vi "Main.vi"() -> ()   [LabVIEW 2025, in "IT-M3900C.lvlib"]
uses:
  IT-M3900C.lvlib
  States Enum.ctl
  Data.ctl
  PS Settings Cluster.ctl
panel:
  out "XY Graph":cluster{timestamp[], dbl[]}[](graph)
  in  "Save":bool
  in  "Test Settings":T1
  in  "Supply Settings":T2={"Repeat"=0, "Terminate Type"=0, "Save File"=1, "Type"=0, "Normal Current(A)"=0.0, "Normal Voltage(V)"=0.0} {"Normal Voltage(V)" min=0.0; "Type" items=["Current", "Voltage"]; "Save File" min=1 max=10; "Terminate Type" items=["Normal", "Last", "Off"]; "Repeat" min=0}
  in  "Current Setpoint":dbl format="%#_g A"
  in  "Set":bool
  in  "Voltage Setpoint":dbl format="%#_g V"
  in  "Enable":bool
  in  "Run":bool
  in  "COM Port":refnum<visa-resource-name>
  out "error out":errorcluster
  in  "error in":errorcluster
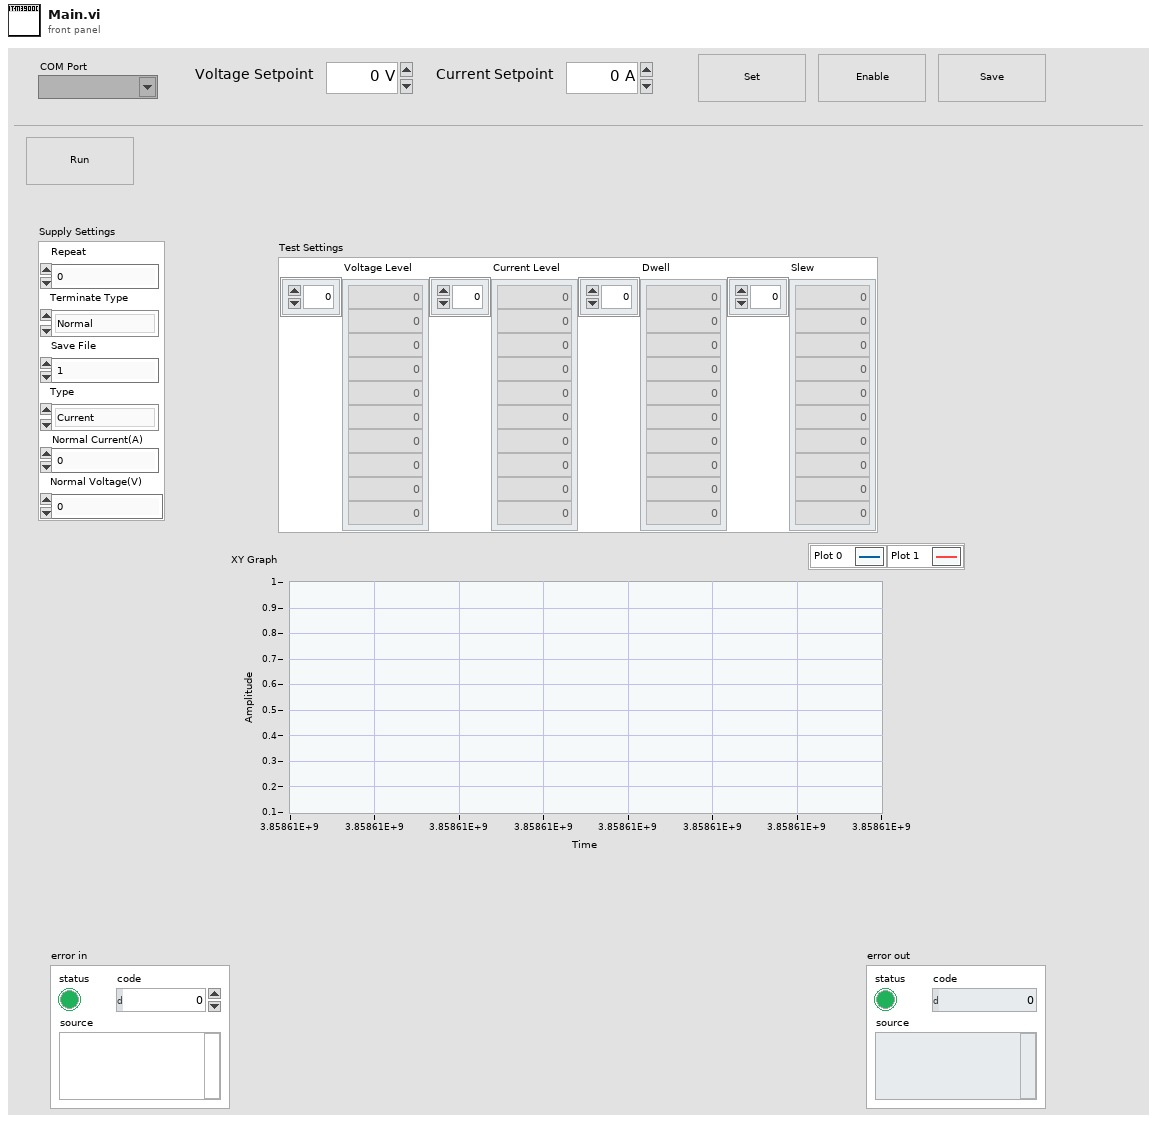
[diagram p1: front panel]
types:
  T1 = cluster{"Voltage Level":dbl[], "Current Level":dbl[], "Dwell":dbl[], "Slew":dbl[]}
  T2 = cluster{"Repeat":i32, "Terminate Type":u16, "Save File":i32, "Type":u16, "Normal Current(A)":dbl, "Normal Voltage(V)":dbl}
  T3 = typedef "IT-M3900C.lvlib/Data.ctl" = cluster{"PS Settings":T4, "Reports Ref":refnum<file>, "Test Settings Ref":refnum<file>, "Test Settings":cluster{"Voltage Level":dbl[], "Current Level":dbl[], "Dwell":dbl[], "Slew":dbl[]}}
  T4 = typedef "IT-M3900C.lvlib/PS Settings Cluster.ctl" = cluster{"COM Port":refnum<visa-resource-name>, "IT Ref":refnum<visa-resource-name>}
  T5 = typedef "IT-M3900C.lvlib/States Enum.ctl" = enum16{"Initialize", "Idle", "Prep Test", "Run", "Wait for Run", "Results", "Exit"}
  T6 = cluster{"Baud Rate":u32, "Parity":u16, "Data Bits":u16, "Stop Bits":u16, "Flow Control":u16}
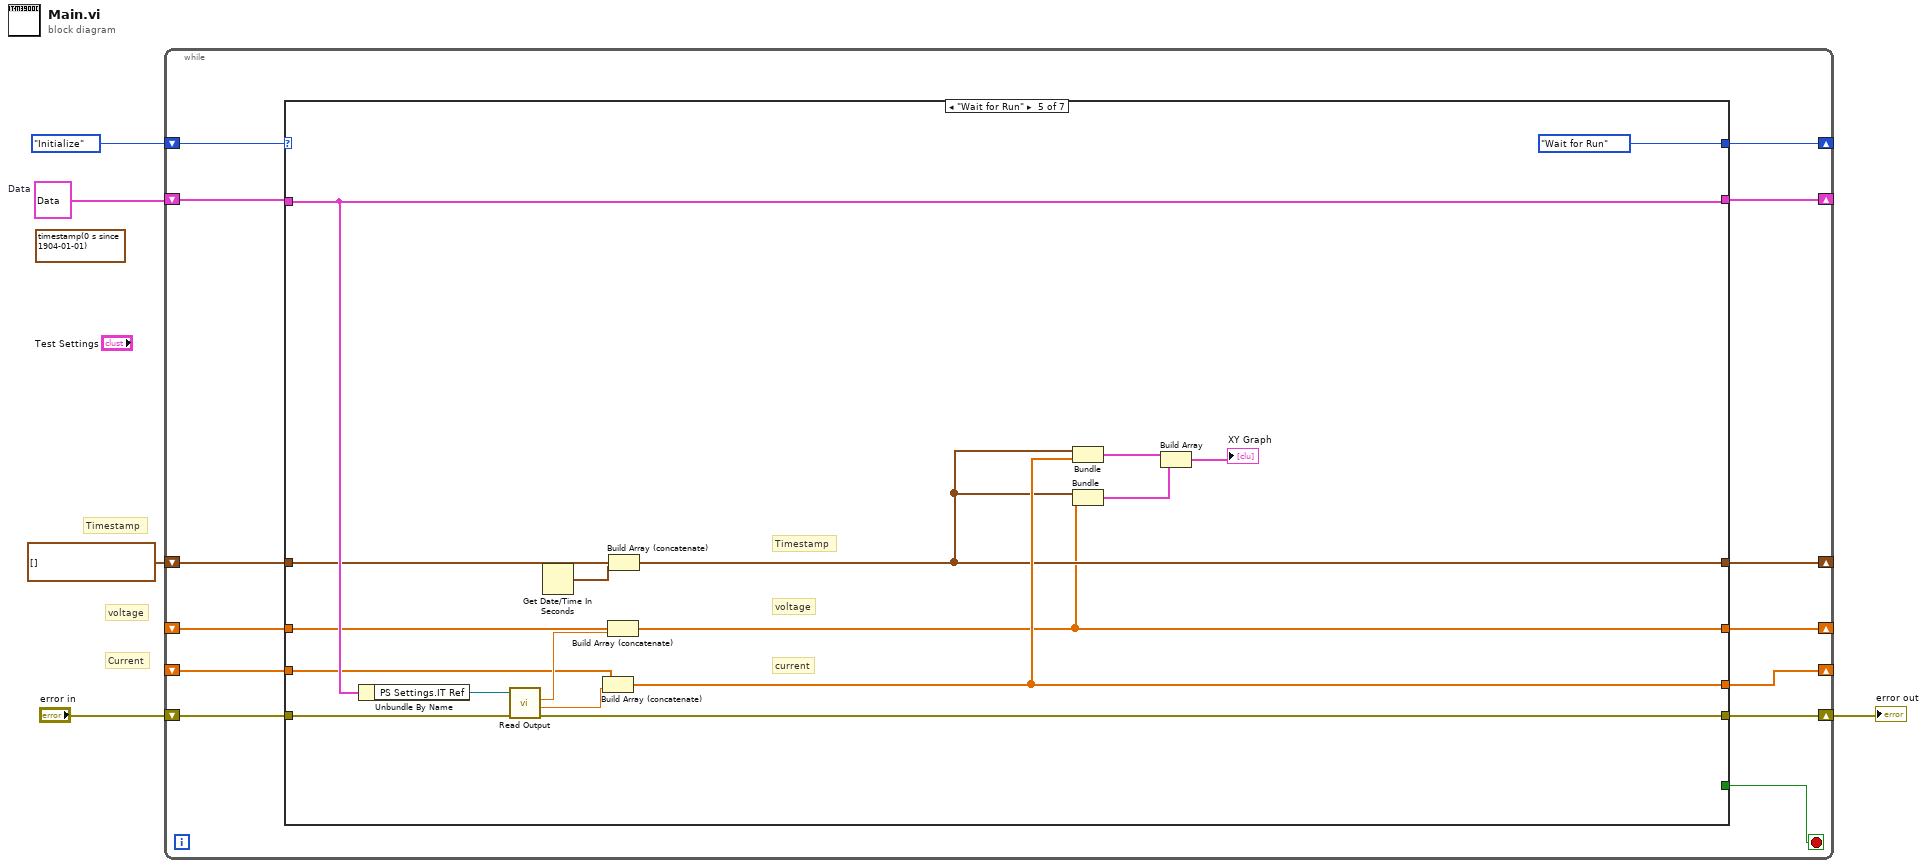
[diagram p0: block diagram]
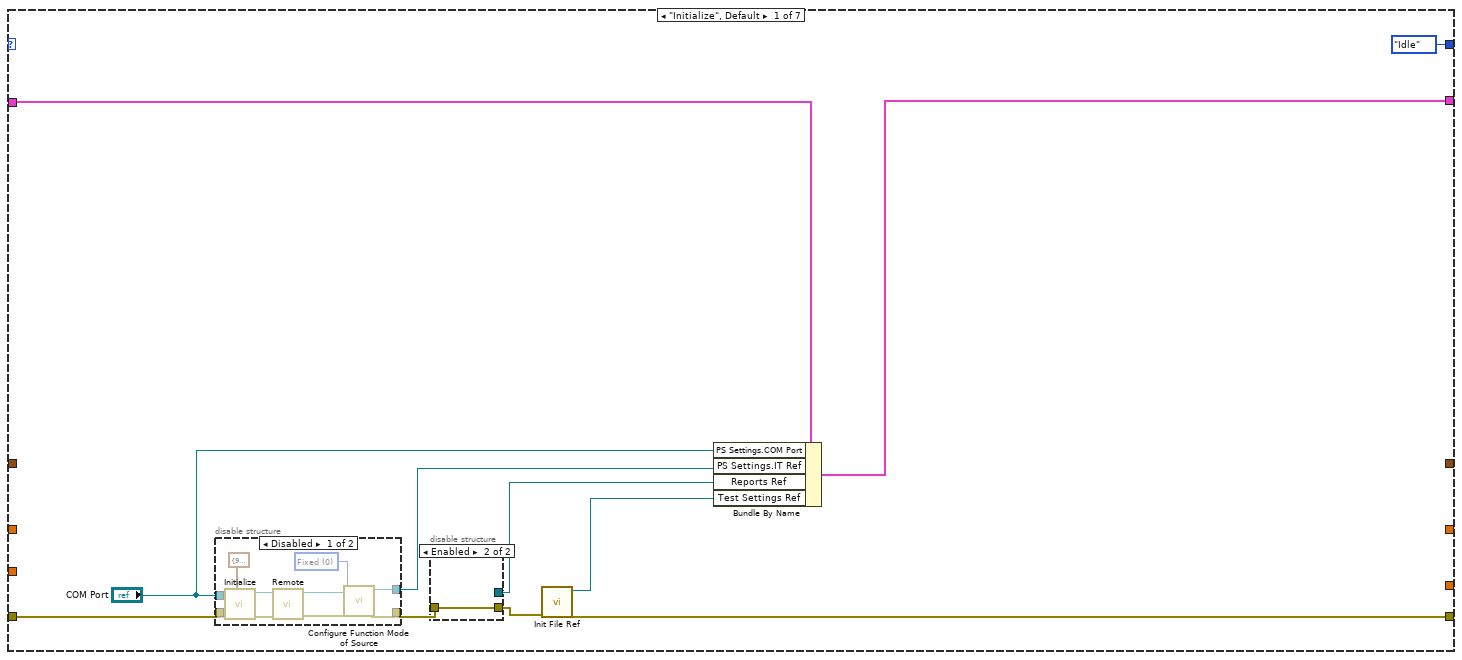
[diagram p2: hidden frame]
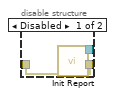
[diagram p3: hidden frame]
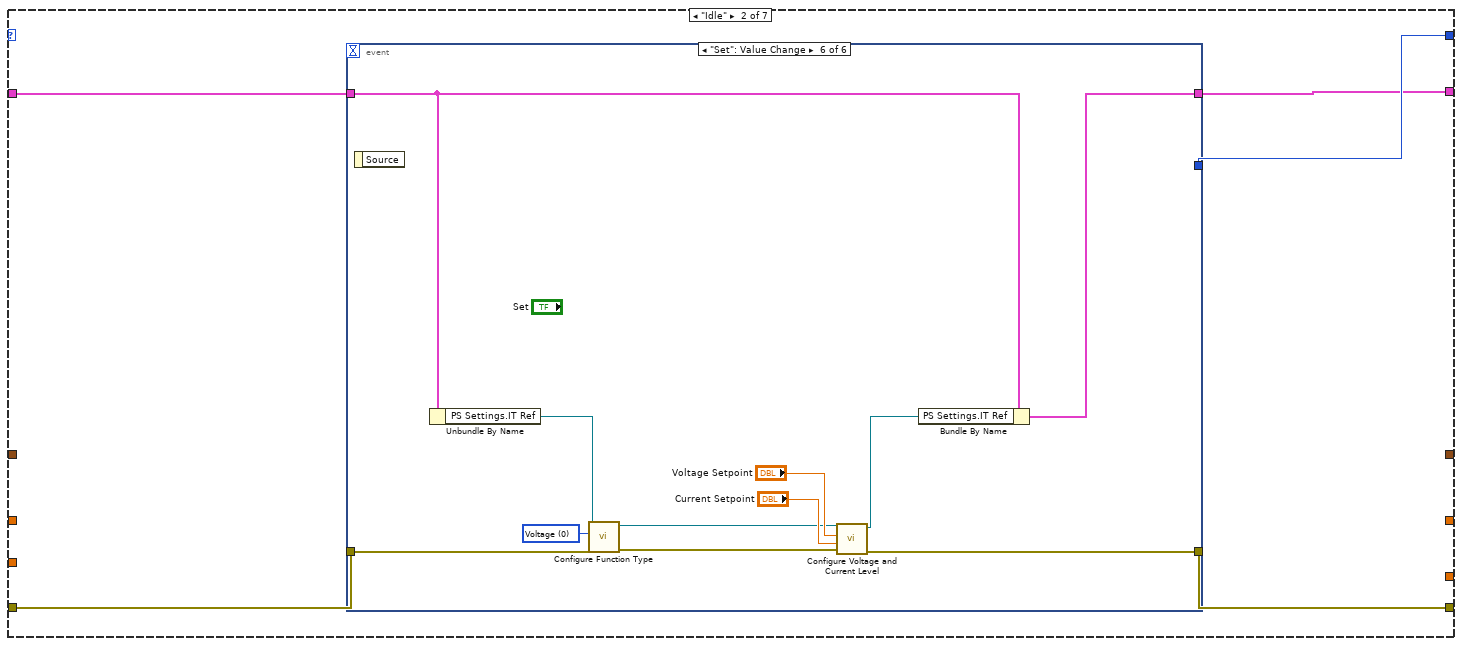
[diagram p5: hidden frame]
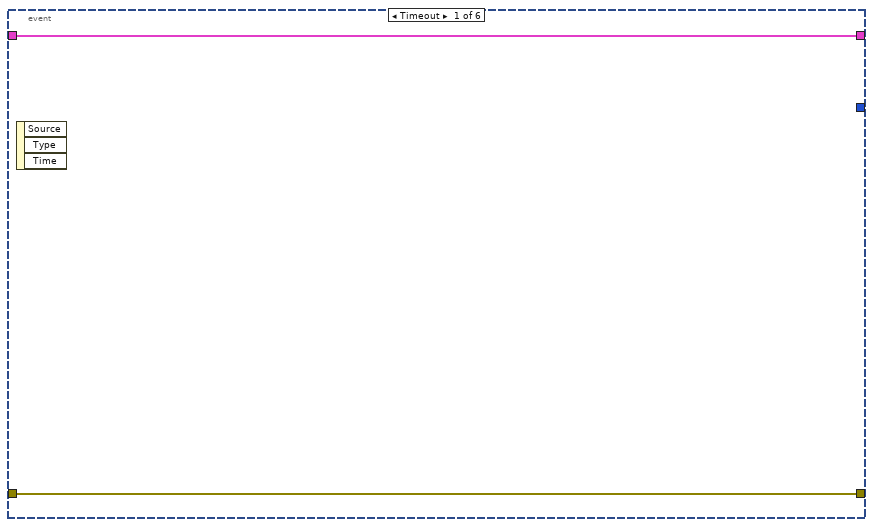
[diagram p6: hidden frame]
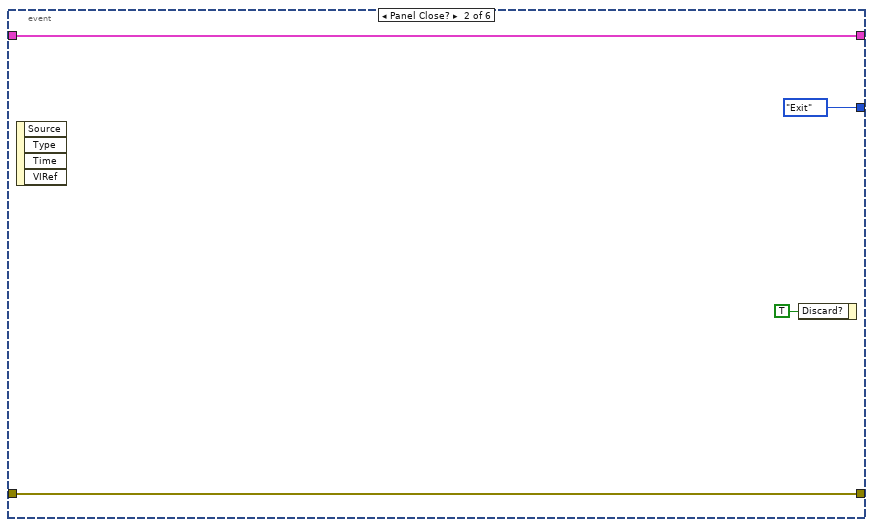
[diagram p7: hidden frame]
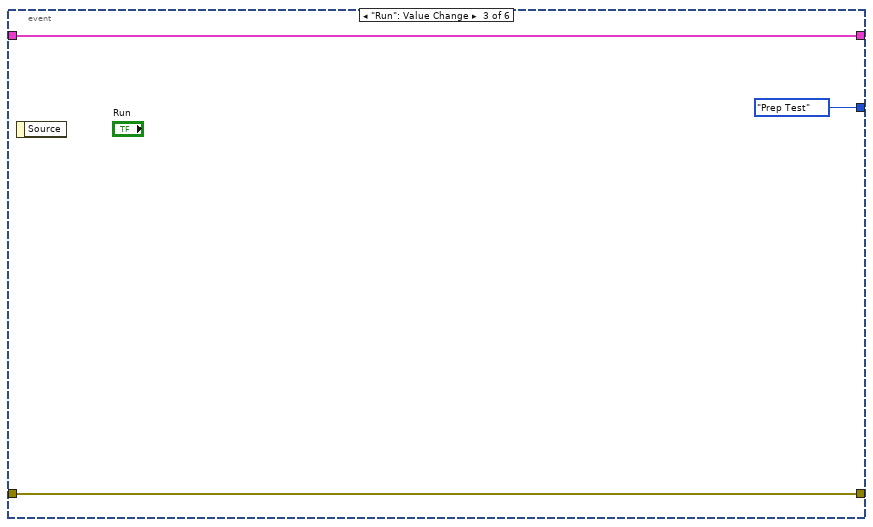
[diagram p8: hidden frame]
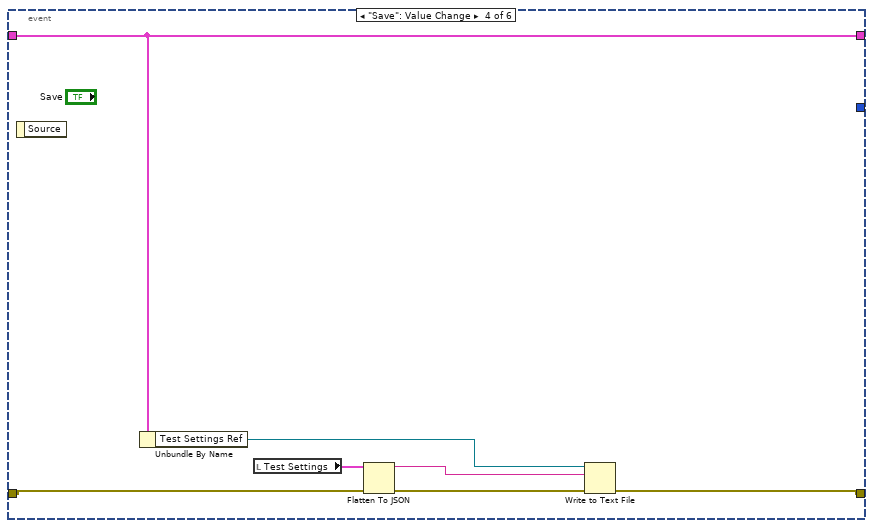
[diagram p9: hidden frame]
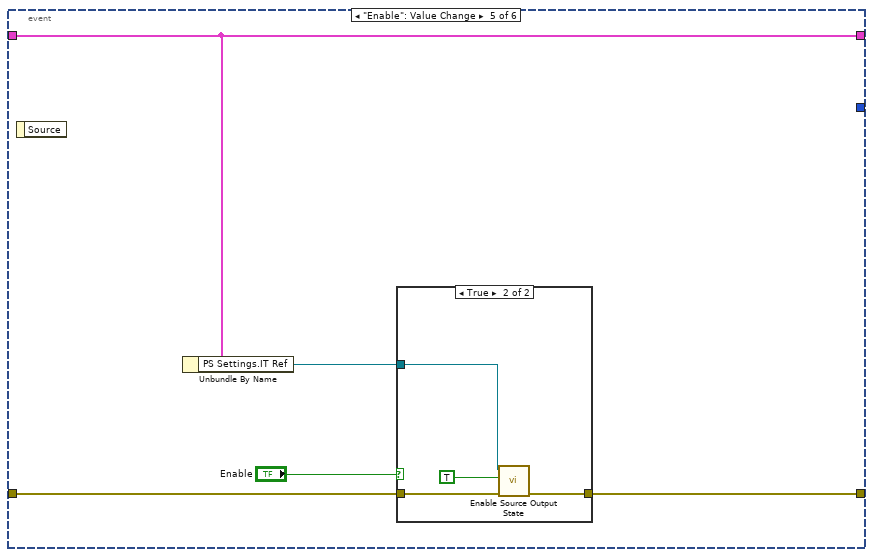
[diagram p10: hidden frame]
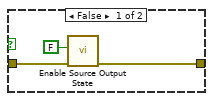
[diagram p11: hidden frame]
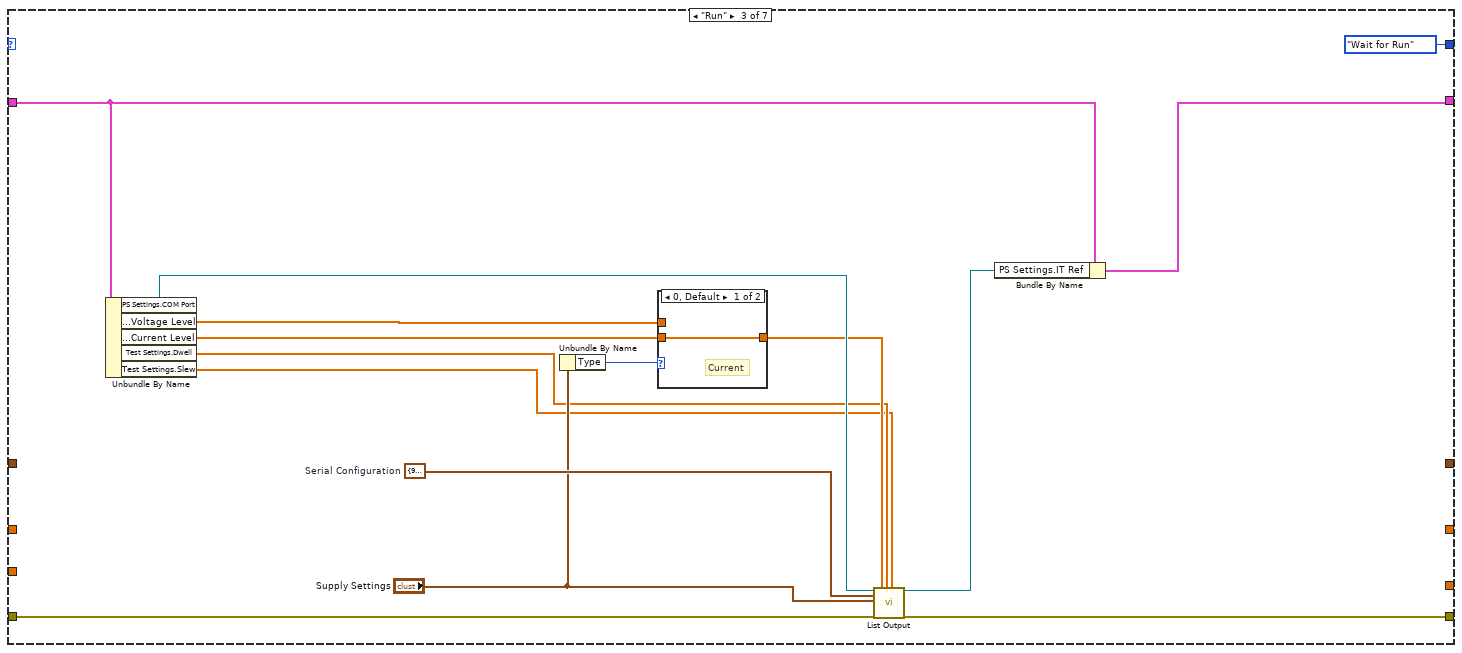
[diagram p12: hidden frame]
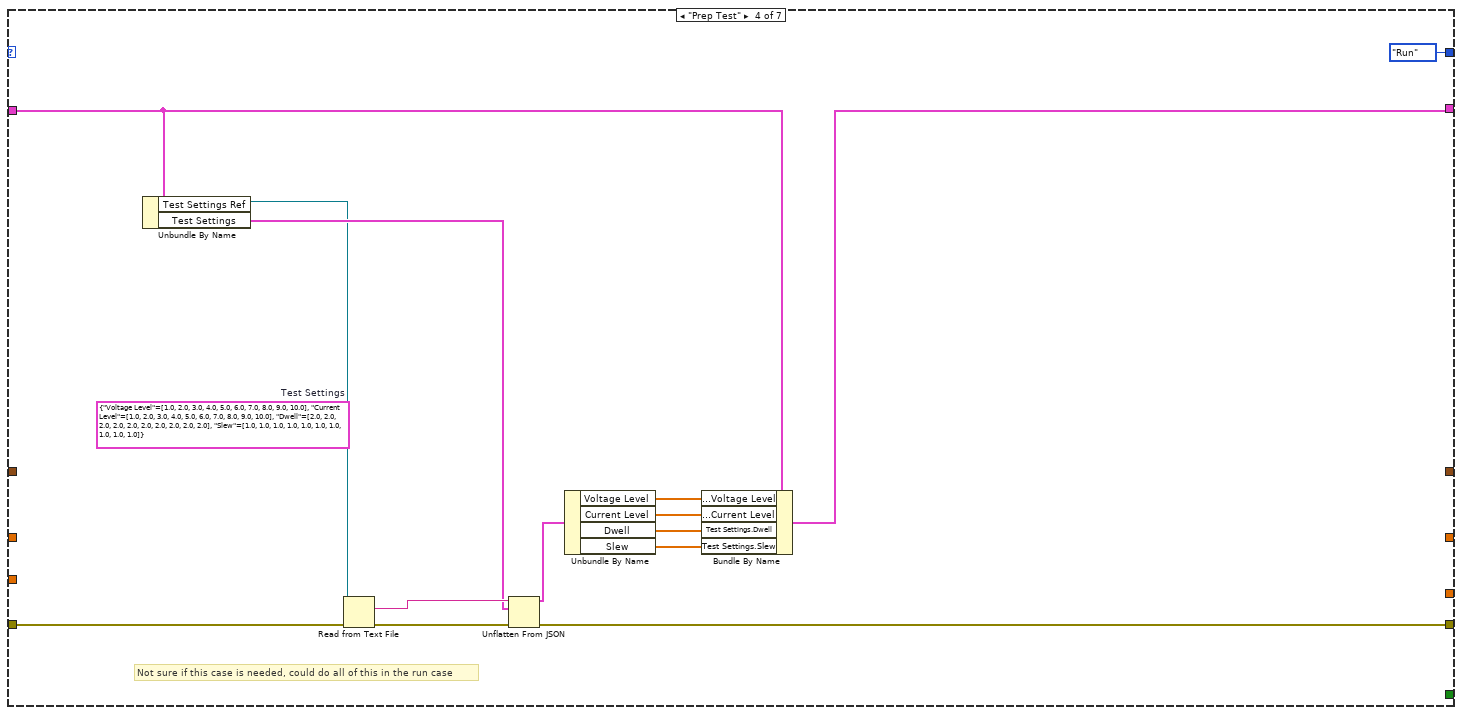
[diagram p14: hidden frame]
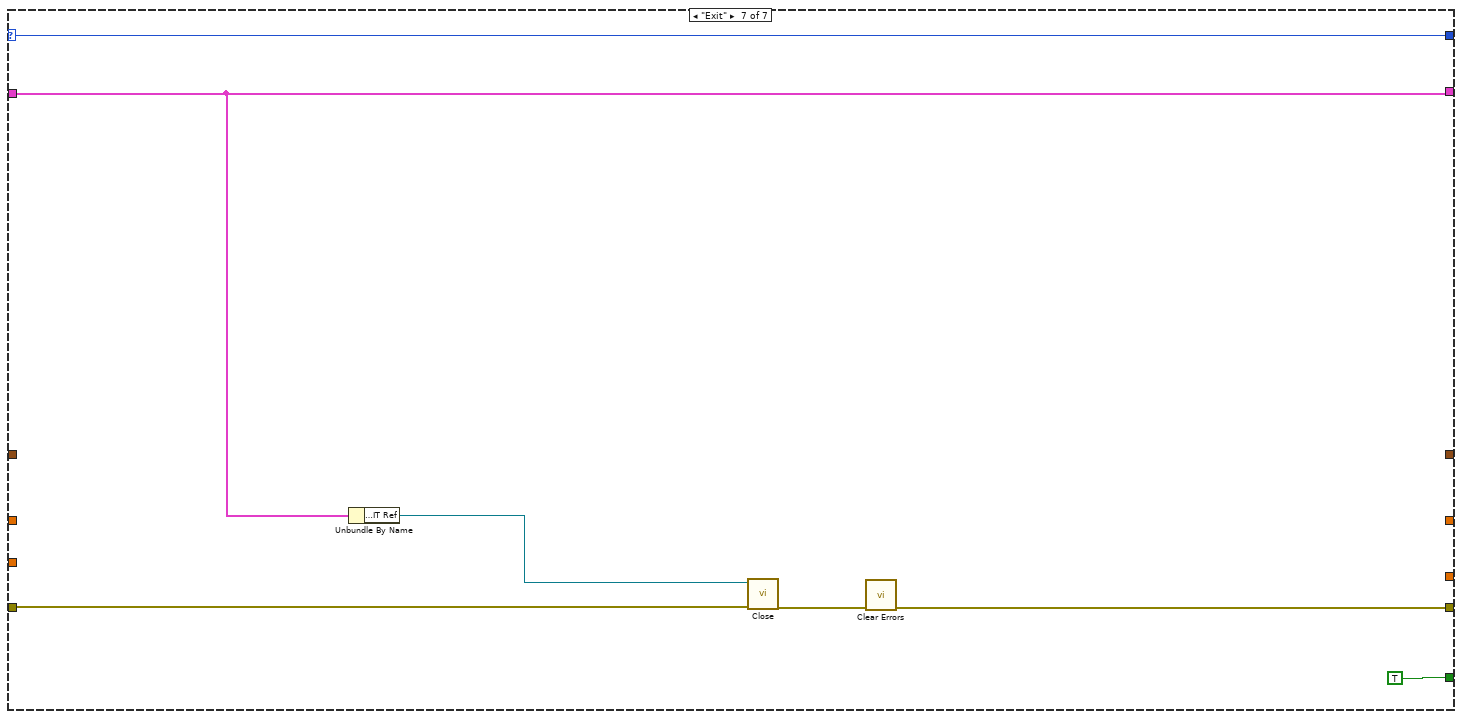
[diagram p16: hidden frame]
diagram:
  (unwired) timestamp(0 s since 1904-01-01) ("seconds since 1Jan1904")
  w2 = T3 {"PS Settings"={"COM Port"="", "IT Ref"=""}, "Reports Ref"=refnum, "Test Settings Ref"=refnum, "Test Settings"={"Voltage Level"=[], "Current Level"=[], "Dwell"=[], "Slew"=[]}}  # Data
  # "Current"
  # "Timestamp"
  # "voltage"
  n1 = while {
    shift-right: [w17] -> _
    shift-left: States_Enum."Initialize" ("States") -> [w18]
    shift-right: [w14] -> w3
    shift-left: "error in" -> [w15]
    shift-right: [w13] -> _
    shift-left: w2 -> [w12]
    shift-right: [w11] -> _
    shift-left: _ -> [w10]
    shift-right: [w9] -> _
    shift-left: timestamp[] [] -> [w8]
    shift-right: [w7] -> _
    shift-left: _ -> [w6]
    stop <- w16 stop-if-true
    n2 = case shown="\"Wait for Run\"" w18 {
      selector: w18 -> [_ _ _ _ _ _ w145]
      tunnel: [States_Enum."Idle" ("States") w48 States_Enum."Wait for Run" ("States") States_Enum."Run" ("States") States_Enum."Wait for Run" ("States") _ w145] -> w17
      tunnel: [_ _ _ _ _ _ TRUE] -> w16
      tunnel: w15 -> [w26 w49 w103 w118 w136 w138 w141]
      tunnel: [w25 w45 w102 w116 w135 w138 w139] -> w14
      tunnel: w12 -> [w29 w47 w90 w112 w134 w137 w143]
      tunnel: [w28 w46 w91 w113 w134 w137 w143] -> w13
      tunnel: [_ _ _ _ w123 _ _] -> w11
      tunnel: w10 -> [_ _ _ _ w131 _ _]
      tunnel: [_ _ _ _ w124 _ _] -> w9
      tunnel: w8 -> [_ _ _ _ w129 _ _]
      tunnel: [_ _ _ _ w126 _ _] -> w7
      tunnel: w6 -> [_ _ _ _ w127 _ _]
      frame "Initialize", Default {
        n3 = disable-structure shown="Disabled" {
          disable-tunnel: w26 -> [w43 w44]
          disable-tunnel: [w39 w44] -> w23
          disable-tunnel: [w37 _] -> w22
          disable-tunnel: "COM Port" -> [w34 _]
          frame Disabled {
            w36 = u16 0 items=["Fixed", "List", "Battery", "Solar", "CarProfile", "Fuel", "Step"] ("Mode")
            n4 = call "Initialize.vi"("Serial Configuration"=T6 {"Baud Rate"=9600, "Parity"=0, "Data Bits"=8, "Stop Bits"=10, "Flow Control"=0}, "error in"=w43, "VISA resource name"=w34) -> ("error out"=w42:errorcluster, "VISA resource name out"=w41:refnum<visa-resource-name>)  [unwired: 7 in]
            n5 = call "Remote.vi"("error in"=w42, "VISA resource name"=w41) -> ("error out"=w40:errorcluster, "VISA resource name out"=w38:refnum<visa-resource-name>)  [unwired: 8 in]
            n6 = call "Configure Function Mode of Source.vi"("error in"=w40, "Mode"=w36, "VISA resource name"=w38) -> ("error out"=w39:errorcluster, "VISA resource name out"=w37:refnum<visa-resource-name>)  [unwired: 7 in]
          }
          frame Enabled {
          }
        }
        n7 = disable-structure shown="Enabled" {
          disable-tunnel: [w32 _] -> w24
          disable-tunnel: w23 -> [w31 w33]
          disable-tunnel: [w30 w33] -> w21
          frame Disabled {
            n8 = call "Init Report.vi"("error in"=w31) -> ("error out"=w30:errorcluster, "Reports"=w32:refnum<file>)  [unwired: 9 in]
          }
          frame Enabled {
          }
        }
        n9 = call "Init File Ref.vi"("error in"=w21) -> ("error out"=w25:errorcluster, "Test Settings"=w20:refnum<file>)  [unwired: 9 in]
        n10 = Bundle By Name(cluster=w29, "PS Settings.COM Port"="COM Port", "PS Settings.IT Ref"=w22, "Reports Ref"=w24, "Test Settings Ref"=w20) -> (w28:T3)
      }
      frame "Idle" {
        n11 = event shown="[5] \"Set\": Value Change" {
          selector: _ -> [_ _ _ _ _ _]
          dyn-events: _ -> [_ _ _ _ _ _]
          timeout: _ -> [_ _ _ _ _ _]
          tunnel: w49 -> [w51 w54 w57 w65 w70 w82]
          tunnel: [_ States_Enum."Exit" ("States") States_Enum."Prep Test" ("States") _ _ _] -> w48
          tunnel: w47 -> [w50 w52 w56 w59 w67 w83]
          tunnel: [w50 w52 w56 w59 w67 w84] -> w46
          tunnel: [w51 w54 w57 w63 w69 w88] -> w45
          event Timeout {
            n12 = event-data() -> ()  [unwired: 1 in, 3 out]
          }
          event Panel Close? {
            n13 = event-data() -> ()  [unwired: 1 in, 4 out]
            n14 = event-data("Discard?"=TRUE) -> ()  [unwired: 1 in, 1 out]
          }
          event "Run": Value Change {
            n15 = event-data() -> ()  [unwired: 1 in, 1 out]
          }
          event "Save": Value Change {
            n16 = event-data() -> ()  [unwired: 1 in, 1 out]
            n17 = Unbundle By Name(w59) -> ("Test Settings Ref"=w61:refnum<file>)
            n18 = local read "Test Settings"() -> (w64:T1)
            n19 = Flatten To JSON(anything=w64, error in (no error)=w65) -> (JSON string=w62:string, 11:w60:errorcluster)  [unwired: 1 in]
            n20 = Write to Text File(file (use dialog)=w61, text=w62, error in=w60) -> (error out=w63:errorcluster)  [unwired: 1 in, 2 out]
          }
          event "Enable": Value Change {
            n21 = event-data() -> ()  [unwired: 1 in, 1 out]
            n22 = Unbundle By Name(w67) -> ("PS Settings.IT Ref"=w66:refnum<visa-resource-name>)
            n23 = case shown="True" "Enable" {
              tunnel: w70 -> [w73 w77]
              tunnel: [w72 w76] -> w69
              tunnel: w66 -> [_ w74]
              frame False {
                n24 = call "Enable Source Output State.vi"("error in"=w73, "State"=FALSE) -> ("error out"=w72:errorcluster)  [unwired: 8 in, 1 out]
              }
              frame True {
                n25 = call "Enable Source Output State.vi"("error in"=w77, "State"=TRUE, "VISA resource name"=w74) -> ("error out"=w76:errorcluster)  [unwired: 7 in, 1 out]
              }
            }
          }
          event "Set": Value Change {
            w78 = u16 0 items=["Voltage", "Current"] ("Type")
            n26 = event-data() -> ()  [unwired: 1 in, 1 out]
            n27 = Unbundle By Name(w83) -> ("PS Settings.IT Ref"=w80:refnum<visa-resource-name>)
            n28 = call "Configure Function Type.vi"("error in"=w82, "Type"=w78, "VISA resource name"=w80) -> ("error out"=w81:errorcluster, "VISA resource name out"=w79:refnum<visa-resource-name>)  [unwired: 7 in]
            n29 = call "Configure Voltage and Current Level.vi"("error in"=w81, "Current(A)"="Current Setpoint", "Voltage(V)"="Voltage Setpoint", "VISA resource name"=w79) -> ("error out"=w88:errorcluster, "VISA resource name out"=w85:refnum<visa-resource-name>)  [unwired: 6 in]
            n30 = Bundle By Name(cluster=w83, "PS Settings.IT Ref"=w85) -> (w84:T3)
          }
        }
      }
      frame "Run" {
        w100 = T6 {"Baud Rate"=9600, "Parity"=0, "Data Bits"=8, "Stop Bits"=10, "Flow Control"=0}  # Serial Configuration
        n31 = Unbundle By Name(w90) -> ("PS Settings.COM Port"=w101:refnum<visa-resource-name>, "Test Settings.Voltage Level"=w97:dbl[], "Test Settings.Current Level"=w96:dbl[], "Test Settings.Dwell"=w94:dbl[], "Test Settings.Slew"=w93:dbl[])
        n32 = Unbundle By Name("Supply Settings") -> ("Type"=w98:u16)
        n33 = case shown="0, Default" w98 {
          tunnel: w97 -> [_ w105]
          tunnel: w96 -> [w104 _]
          tunnel: [w104 w105] -> w95
          frame 0, Default {
            # "Current"
          }
          frame 1 {
            # "Voltage"
          }
        }
        n34 = call "List Output.vi"("VISA resource name"=w101, "Serial Configuration"=w100, "Supply Settings"="Supply Settings", "error in"=w103, "Level(V/A/W/ohm)"=w95, "Dwell(S)"=w94, "Slew"=w93) -> ("VISA resource name out"=w89:refnum<visa-resource-name>, "error out"=w102:errorcluster)  [unwired: 11 in]
        n35 = Bundle By Name(cluster=w90, "PS Settings.IT Ref"=w89) -> (w91:T3)
      }
      frame "Prep Test" {
        (unwired) T1 {"Voltage Level"=[1.0, 2.0, 3.0, 4.0, 5.0, 6.0, 7.0, 8.0, 9.0, 10.0], "Current Level"=[1.0, 2.0, 3.0, 4.0, 5.0, 6.0, 7.0, 8.0, 9.0, 10.0], "Dwell"=[2.0, 2.0, 2.0, 2.0, 2.0, 2.0, 2.0, 2.0, 2.0, 2.0], "Slew"=[1.0, 1.0, 1.0, 1.0, 1.0, 1.0, 1.0, 1.0, 1.0, 1.0]}  # Test Settings
        # "Not sure if this case is needed, could do all of this in the run case"
        n36 = Unbundle By Name(w112) -> ("Test Settings Ref"=w106:refnum<file>, "Test Settings"=w107:T1)
        n37 = Read from Text File(file (use dialog)=w106, error in=w118) -> (text=w115:string, error out=w117:errorcluster)  [unwired: 2 in, 2 out]
        n38 = Unflatten From JSON(JSON string=w115, type and defaults=w107, error in (no error)=w117) -> (value=w114:T1, error out=w116:errorcluster)  [unwired: 4 in]
        n39 = Unbundle By Name(w114) -> ("Voltage Level"=w111:dbl[], "Current Level"=w110:dbl[], "Dwell"=w109:dbl[], "Slew"=w108:dbl[])
        n40 = Bundle By Name(cluster=w112, "Test Settings.Voltage Level"=w111, "Test Settings.Current Level"=w110, "Test Settings.Dwell"=w109, "Test Settings.Slew"=w108) -> (w113:T3)
      }
      frame "Wait for Run" {
        # "Timestamp"
        # "current"
        # "voltage"
        n41 = Unbundle By Name(w134) -> ("PS Settings.IT Ref"=w133:refnum<visa-resource-name>)
        n42 = call "Read Output.vi"("error in"=w136, "VISA resource name"=w133) -> ("error out"=w135:errorcluster, "Actual Current Level (A)"=w128:dbl, "Actual Voltage Level (V)"=w132:dbl)  [unwired: 6 in, 1 out]
        n43 = Get Date/Time In Seconds() -> (seconds since 1Jan1904=w130:timestamp)
        n44 = Build Array (concatenate)(w127, w128) -> (w126:dbl[])
        n45 = Build Array (concatenate)(w131, w132) -> (w123:dbl[])
        n46 = Build Array (concatenate)(w129, w130) -> (w124:timestamp[])
        n47 = Bundle(w124, w126) -> (w122:cluster{timestamp[], dbl[]})  [unwired: 1 in]
        n48 = Bundle(w124, w123) -> (w121:cluster{timestamp[], dbl[]})  [unwired: 1 in]
        n49 = Build Array(w122, w121) -> (→"XY Graph":cluster{timestamp[], dbl[]}[])
      }
      frame "Results" {
      }
      frame "Exit" {
        n50 = Unbundle By Name(w143) -> ("PS Settings.IT Ref"=w142:refnum<visa-resource-name>)
        n51 = call "Close.vi"("error in"=w141, "VISA resource name"=w142) -> ("error out"=w140:errorcluster)  [unwired: 9 in]
        n52 = call <vilib>:"Clear Errors.vi"("error in (no error)"=w140) -> ("error out"=w139:errorcluster)  [unwired: 5 in, 1 out]
      }
    }
  }
  "error out" <- w3
